vi "Teleop DriveForward.vi"(8 "error in":errorcluster, 11 "Data Input":T1) -> (0 "error out":errorcluster, 3 "Data Output":T1)   [LabVIEW 2018]
uses:
  TypeDefs/Teleop Data Cluster.ctl
  TypeDefs/Joystick Axes.ctl
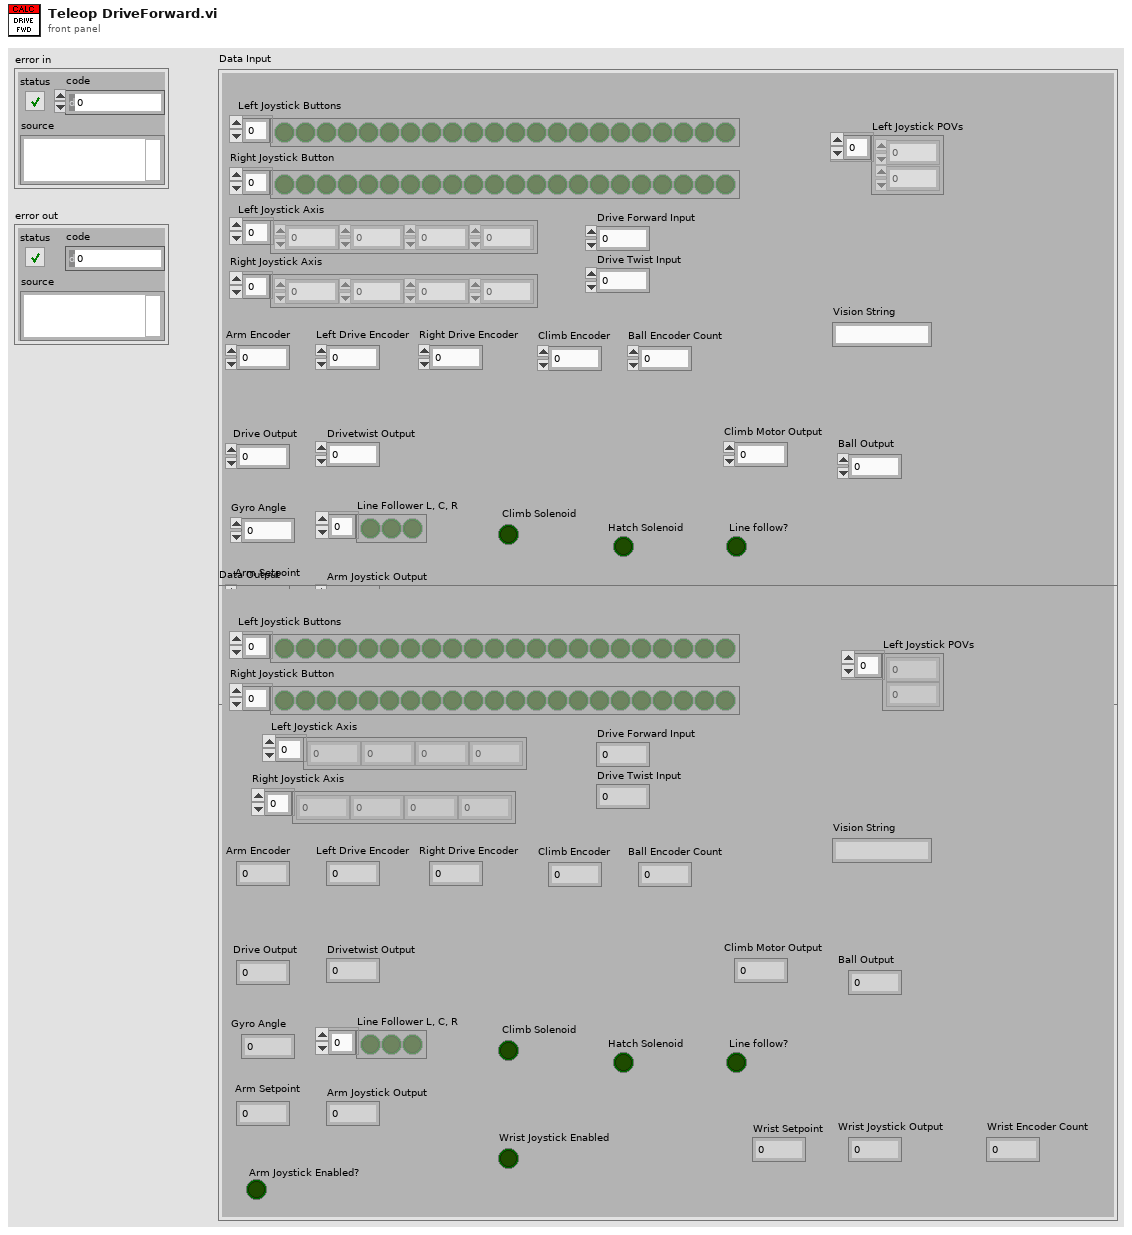
[diagram p1: front panel]
types:
  T1 = typedef "Teleop Data Cluster.ctl" = cluster{"Drive Forward Input ":dbl, "Drive Twist Input":dbl, "Drive Output":dbl, "Drivetwist Output":dbl, "Left Joystick Buttons":bool[], "Left Joystick Axis":dbl[], "Right Joystick Axis":dbl[], "Right Joystick Button":bool[], "Arm Encoder":dbl, "Left Drive Encoder":dbl, "Right Drive Encoder":dbl, "Gyro Angle ":dbl, "Arm Joystick Output  ":dbl, "Line Follower L, C, R ":bool[], "Line follow?":bool, " Climb Solenoid":bool, "Wrist Encoder Count":dbl, "Wrist Joystick Output":dbl, "Ball Encoder Count":dbl, "Ball Output":dbl, "Climb Encoder":dbl, "Climb Motor Output":dbl, " Hatch Solenoid":bool, "Arm Setpoint ":dbl, "Wrist Setpoint ":dbl, "Arm Joystick Enabled?":bool, "Wrist Joystick Enabled":bool, "Vision String":string, "Left Joystick POVs":i16[]}
  T2 = typedef "Joystick Axes.ctl" = enum16{"X Axis", "Y Axis", "Twist Axis", "Throttle"}
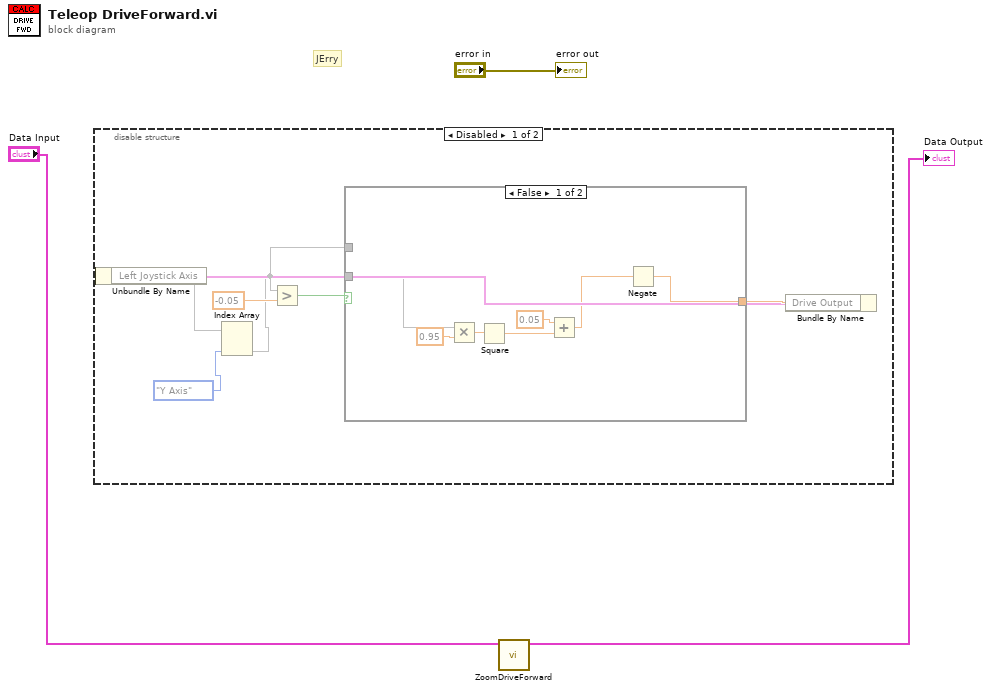
[diagram p0: block diagram]
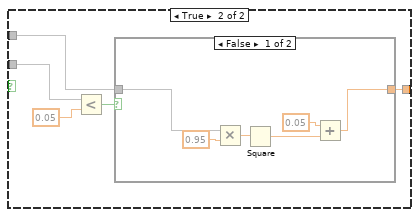
[diagram p2: hidden frame]
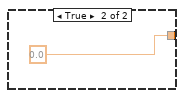
[diagram p3: hidden frame]
diagram:
  # "JErry"
  n1 = disable-structure shown="Disabled" {
    frame Disabled {
      n2 = Unbundle By Name(w8) -> ("Left Joystick Axis"=w6)
      n3 = Index Array(array=w6, index #2=Joystick_Axes."Y Axis" ("Enum")) -> (element #2=w5)  [unwired: 1 in, 1 out]
      n4 = Greater?(x=w5, y=-0.05) -> (0:w11:bool)
      n5 = case shown="False" w11 {
        tunnel: w5 -> [w17 w19]
        tunnel: [w18 w21] -> w9
        tunnel: w5 -> [_ w20]
        frame False {
          n6 = Multiply(x=w17, y=0.95) -> (x*y=w15:dbl)
          n7 = Square(x=w15) -> (x^2=w14:dbl)
          n8 = Add(x=0.05, y=w14) -> (x+y=w12:dbl)
          n9 = Negate(x=w12) -> (-x=w18:dbl)
        }
        frame True {
          n10 = Less?(x=w19, y=0.05) -> (x < y?=w23:bool)
          n11 = case shown="False" w23 {
            tunnel: [w24 0.0] -> w21
            tunnel: w20 -> [w25 _]
            frame False {
              n12 = Multiply(x=w25, y=0.95) -> (x*y=w28:dbl)
              n13 = Square(x=w28) -> (x^2=w27:dbl)
              n14 = Add(x=0.05, y=w27) -> (x+y=w24:dbl)
            }
            frame True {
            }
          }
        }
      }
      n15 = Bundle By Name("Drive Output"=w9) -> (w7:cluster{}, w8:cluster{})
    }
    frame Enabled {
    }
  }
  n16 = call "ZoomDriveForward.vi"("Cluster In"="Data Input") -> ("Cluster Out"=→"Data Output":T1)  [unwired: 10 in]
  "error out" <- "error in"
